vi "PowerUp Old.vi"(0 "Voltage Level DxSupply":dbl, 1 "Current Limit  DxBoot0":dbl, 2 "Voltage Level DxBoot0":dbl, 3 "FPGA Reference In":refnum<k20>, 5 "Current Limit DxSupply":dbl, 7 "DxBoot0":string="0", 9 "DxSupply":string="0", 11 "error in (no error)":errorcluster, 12 "SMU Handle":refnum<k15>="PXI1Slot2", 13 "nReset Task":refnum<k21>, 14 "Reset Pulse Time (ms)":dbl) -> (15 "error out":errorcluster)   [LabVIEW 2018]
uses:
  Resources_Test/UART/ControlTestSlot.ctl
  <vilib>/DAQmx/write.llb/DAQmx Write (Digital Bool 1Line 1Point).vi
  <vilib>/DAQmx/miscellaneous.llb/DAQmx Fill In Error Info.vi
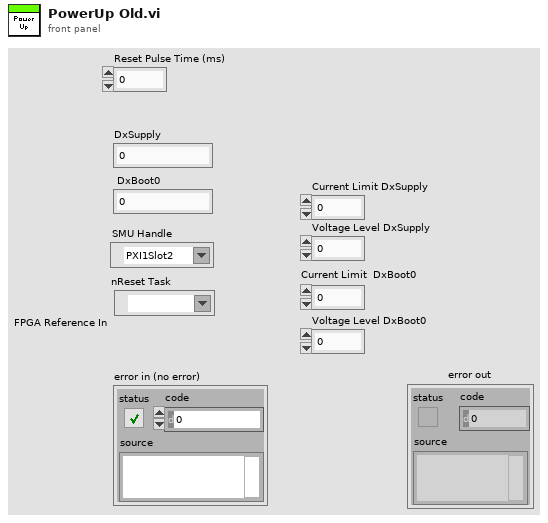
[diagram p1: front panel]
types:
  T1 = typedef "ControlTestSlot.ctl" = enum16{"DUT 1", "DUT 2"}
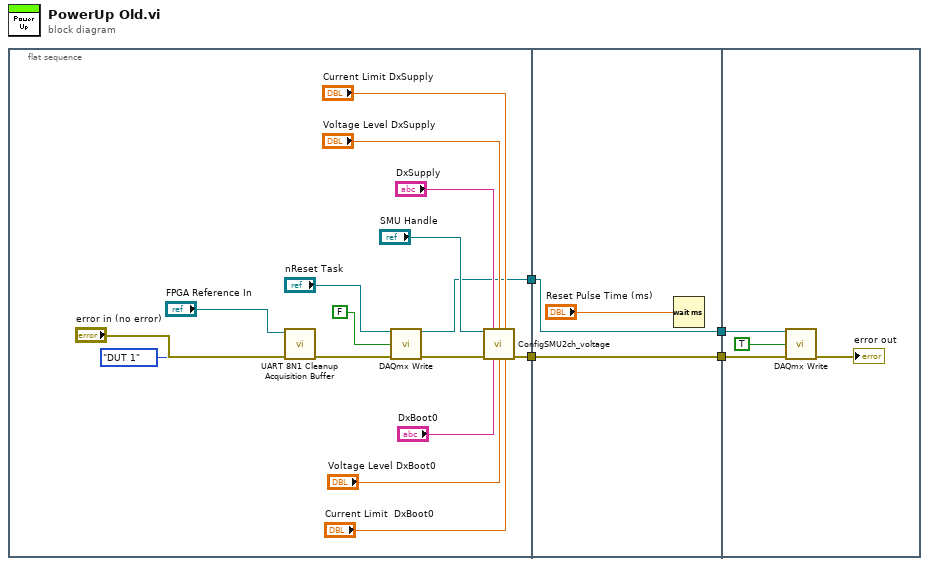
[diagram p0: block diagram]
diagram:
  n1 = flat-sequence {
    tunnel: [w10] -> w3
    tunnel: [w9] -> w1
    tunnel: [w22] -> w4
    tunnel: w3 -> [w22]
    tunnel: [w21] -> w2
    tunnel: w1 -> [w21]
    tunnel: w4 -> [w26]
    tunnel: w2 -> [w24]
    frame #0 {
      n2 = call "UART 8N1 Cleanup Acquisition Buffer.vi"("Error In"="error in (no error)", "Enum"=ControlTestSlot."DUT 1", "FPGA Reference In"="FPGA Reference In") -> ("Error Out"=w7:errorcluster)  [unwired: 7 in, 1 out]
      n3 = call-poly <vilib>:"DAQmx Write.vi"("task/channels in"="nReset Task", "data"=FALSE, "error in"=w7) -> ("task out"=w9:refnum<k21>, "error out"=w20:errorcluster)  [unwired: 10 in, 1 out]
      n4 = call "ConfigSMU2ch_voltage.vi"("IVI Refnum in"="SMU Handle", "Channel DxSupply"="DxSupply", "Voltage Level DxSupply"="Voltage Level DxSupply", "Current Limit DxSupply"="Current Limit DxSupply", "error in (no error)"=w20, "Channel DxBoot0"="DxBoot0", "Voltage Level DxBoot0"="Voltage Level DxBoot0", "Current Limit DxBoot0"="Current Limit  DxBoot0") -> ("error out"=w10:errorcluster)  [unwired: 6 in, 1 out]
    }
    frame #1 {
      n5 = Wait (ms)(milliseconds to wait="Reset Pulse Time (ms)") -> ()  [unwired: 1 out]
    }
    frame #2 {
      n6 = call-poly <vilib>:"DAQmx Write.vi"("task/channels in"=w24, "data"=TRUE, "error in"=w26) -> ("error out"=→"error out":errorcluster)  [unwired: 10 in, 2 out]
    }
  }
